vi "Check Action.vi"(6 "HRS Time":dbl, 7 "Values In":dbl[](array[numeric]), 8 "error in (no error)":errorcluster, 11 "PulsedValve in":refnum<class "PulsedControl.lvclass">) -> (0 "error out":errorcluster, 2 "Actions":T1[](array[typedef]), 3 "PulsedValve out":refnum<class "PulsedControl.lvclass">, 5 "Values":dbl[](array[numeric]))   [LabVIEW 2020, in "VolatusControl.lvlib" / "PulsedControl.lvclass"]
uses:
  PulsedControl.lvclass
  Control Action.ctl
  PulsedControl.lvclass/PulsedControl.ctl
  State.ctl
  Volatus/MessageQ/MessageQ.lvclass
  VolatusControl.lvlib
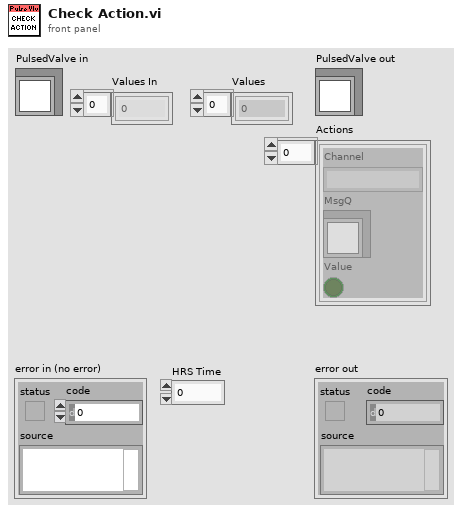
[diagram p1: front panel]
types:
  T1 = typedef "VolatusControl.lvlib/Control Action.ctl" = cluster{"Channel":string, "MsgQ":refnum<class "MessageQ.lvclass">, "Value":bool}
  T2 = typedef "VolatusControl.lvlib/PulsedControl.lvclass/State.ctl" = enum16{"Idle", "Start", "On", "Off"}
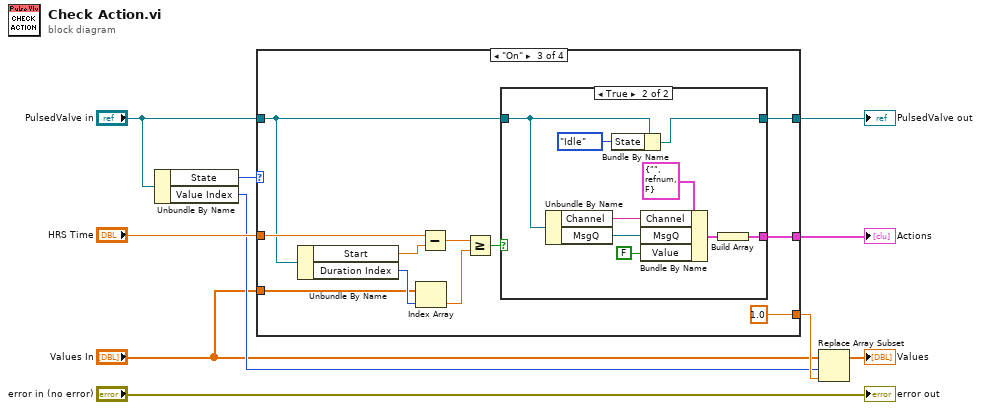
[diagram p0: block diagram]
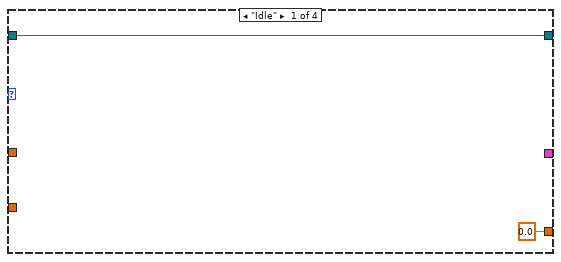
[diagram p2: hidden frame]
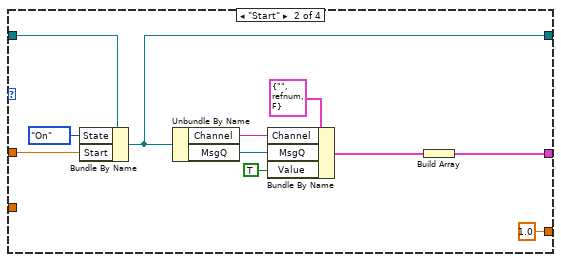
[diagram p3: hidden frame]
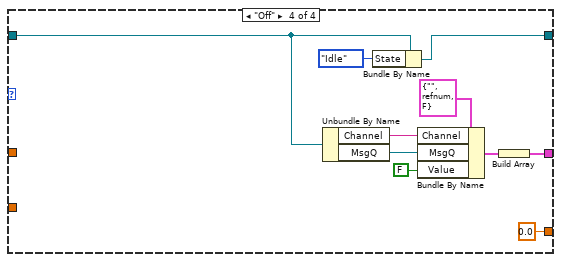
[diagram p5: hidden frame]
diagram:
  n1 = Unbundle By Name("PulsedValve in") -> ("State"=w9:T2, "Value Index"=w2:i32)
  n2 = case shown="\"On\"" w9 {
    tunnel: "HRS Time" -> [_ w23 w34 _]
    tunnel: "PulsedValve in" -> [w12 w21 w29 w49]
    tunnel: [w12 w19 w28 w48] -> w6
    tunnel: [_ w13 w31 w45] -> w5
    tunnel: [0.0 1.0 1.0 0.0] -> w3
    tunnel: "Values In" -> [_ _ w25 _]
    frame "Idle" {
    }
    frame "Start" {
      n3 = Bundle By Name(cluster=w21, "State"=State."On", "Start"=w23) -> (w19:refnum<class "PulsedControl.lvclass">)
      n4 = Unbundle By Name(w19) -> ("Channel"=w17:string, "MsgQ"=w16:refnum<class "MessageQ.lvclass">)
      n5 = Bundle By Name(cluster=T1 {"Channel"="", "MsgQ"=refnum, "Value"=FALSE} ("Action"), "Channel"=w17, "MsgQ"=w16, "Value"=TRUE) -> (w18:T1)
      n6 = Build Array(w18) -> (w13:T1[])
    }
    frame "On" {
      n7 = Unbundle By Name(w29) -> ("Start"=w33:dbl, "Duration Index"=w26:i32)
      n8 = Index Array(array=w25, index=w26) -> (element=w24:dbl)
      n9 = Subtract(x=w34, y=w33) -> (x-y=w32:dbl)
      n10 = Greater Or Equal?(x=w32, y=w24) -> (x >= y?=w30:bool)
      n11 = case shown="True" w30 {
        tunnel: [_ w36] -> w31
        tunnel: w29 -> [w35 w39]
        tunnel: [w35 w37] -> w28
        frame False {
        }
        frame True {
          n12 = Unbundle By Name(w39) -> ("Channel"=w43:string, "MsgQ"=w42:refnum<class "MessageQ.lvclass">)
          n13 = Bundle By Name(cluster=w39, "State"=State."Idle") -> (w37:refnum<class "PulsedControl.lvclass">)
          n14 = Bundle By Name(cluster=T1 {"Channel"="", "MsgQ"=refnum, "Value"=FALSE} ("Action"), "Channel"=w43, "MsgQ"=w42, "Value"=FALSE) -> (w40:T1)
          n15 = Build Array(w40) -> (w36:T1[])
        }
      }
    }
    frame "Off" {
      n16 = Unbundle By Name(w49) -> ("Channel"=w53:string, "MsgQ"=w52:refnum<class "MessageQ.lvclass">)
      n17 = Bundle By Name(cluster=w49, "State"=State."Idle") -> (w48:refnum<class "PulsedControl.lvclass">)
      n18 = Bundle By Name(cluster=T1 {"Channel"="", "MsgQ"=refnum, "Value"=FALSE} ("Action"), "Channel"=w53, "MsgQ"=w52, "Value"=FALSE) -> (w47:T1)
      n19 = Build Array(w47) -> (w45:T1[])
    }
  }
  "PulsedValve out" <- w6
  "Actions" <- w5
  n20 = Replace Array Subset(array="Values In", new element=w3, index=w2) -> (→"Values":dbl[])
  "error out" <- "error in (no error)"
